vi "port to index.vi"(11 "Port":cluster{"module":u8, "channel":u8}) -> (3 "Channel Index":i32)   [LabVIEW 2015]
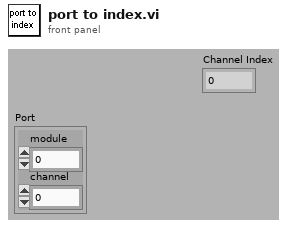
[diagram p1: front panel]
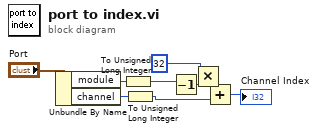
[diagram p0: block diagram]
diagram:
  n1 = Unbundle By Name("Port") -> ("module"=w8:u8, "channel"=w7:u8)
  n2 = To Unsigned Long Integer(number=w8) -> (unsigned 32bit integer=w2:u32)
  n3 = To Unsigned Long Integer(number=w7) -> (unsigned 32bit integer=w1:u32)
  n4 = Decrement(x=w2) -> (x-1=w9:u32)
  n5 = Multiply(x=u8 32, y=w9) -> (x*y=w5:u32)
  n6 = Add(x=w5, y=w1) -> (x+y=→"Channel Index":u32)
